vi "Connect.vi"(8 "error in":errorcluster, 11 "DB-ADO in":refnum<class "DB-ADO.lvclass">) -> (0 "error out":errorcluster, 3 "DB-ADO out":refnum<class "DB-ADO.lvclass">)   [LabVIEW 2022 SP3, in "hse-db-ado.lvlib" / "DB-ADO.lvclass"]
doc: "Connect to a ADO database.\n\n____\nHAMPEL SOFTWARE ENGINEERING v1.4.0 (2023-12-19 09:52)"
uses:
  DB-ADO.lvclass
  C:/Projects/579-Intelligent-Systems-Term-Project/06_Source/UI/FReVSys_Source/Libraries/hse-db/Source/DB-Interface/DB-Interface.lvclass
  DB-Interface/DB-Interface.lvclass/DB-Interface.ctl
  DB-ADO.lvclass/DB-ADO.ctl
  ADO-DB-Drivers/ADO-DB-Driver.lvlib
  DB-Interface/DB-Interface.lvclass
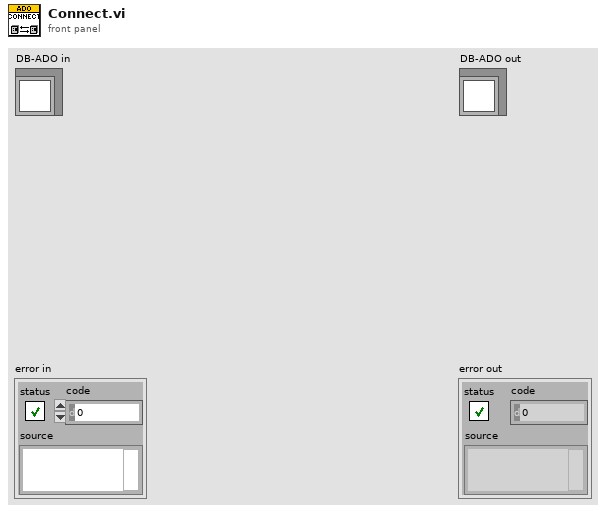
[diagram p1: front panel]
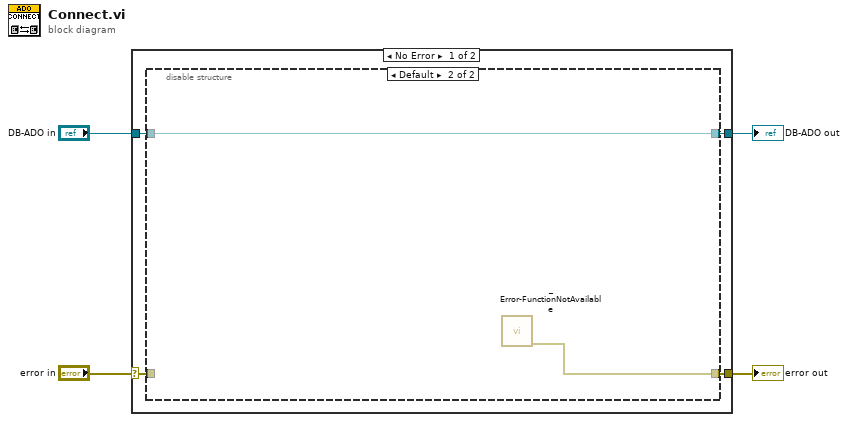
[diagram p0: block diagram]
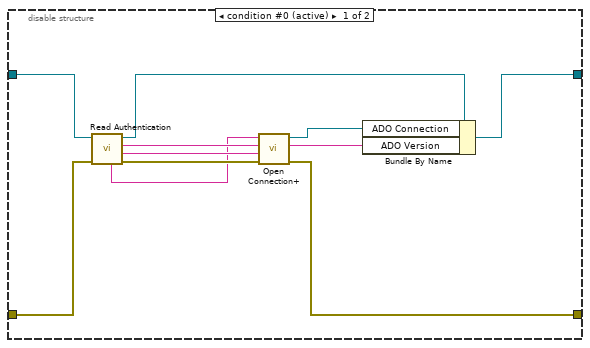
[diagram p2: hidden frame]
diagram:
  n1 = case shown="No Error" "error in" {
    selector: "error in" -> [w7 w23]
    tunnel: [w6 w23] -> w3
    tunnel: [w5 w22] -> w1
    tunnel: "DB-ADO in" -> [w8 w22]
    frame No Error {
      n2 = disable-structure shown="Default" {
        disable-tunnel: w8 -> [w19 w21]
        disable-tunnel: w7 -> [w14 _]
        disable-tunnel: [w13 w20] -> w6
        disable-tunnel: [w10 w21] -> w5
        frame condition #0 (active) {
          n3 = call "Read Authentication.vi"("error in"=w14, "DB-Engine in"=w19) -> ("error out"=w16:errorcluster, "Password"=w17:string, "User"=w18:string, "DB-Engine out"=w11:refnum<class "DB-ADO.lvclass">, "Database"=w15:string)  [unwired: 5 in]
          n4 = call "Open Connection+.vi"("error in (no error)"=w16, "Password"=w17, "UserID"=w18, "Connection String"=w15) -> ("error out"=w13:errorcluster, "ADO Version"=w9:string, "Connection"=w12:refnum<k7>)  [unwired: 5 in]
          n5 = Bundle By Name(cluster=w11, "ADO Connection"=w12, "ADO Version"=w9) -> (w10:refnum<class "DB-ADO.lvclass">)
        }
        frame condition #1 {
          n6 = call "_Error-FunctionNotAvailable.vi"() -> ("error out"=w20:errorcluster)  [unwired: 11 in]
        }
      }
    }
    frame Error {
    }
  }
  "error out" <- w3
  "DB-ADO out" <- w1
